vi "Initialize.vi"(0 "Universal Robot in":refnum<class "Universal Robot.lvclass">, 5 "error in (no error)":errorcluster) -> (14 "Universal Robot out":refnum<class "Universal Robot.lvclass">, 19 "error out":errorcluster)   [LabVIEW 2016, in "Universal Robot.lvclass"]
uses:
  Universal Robot.lvclass
  Universal Robot.lvclass/Universal Robot.ctl
  ProgramControlEvent.ctl
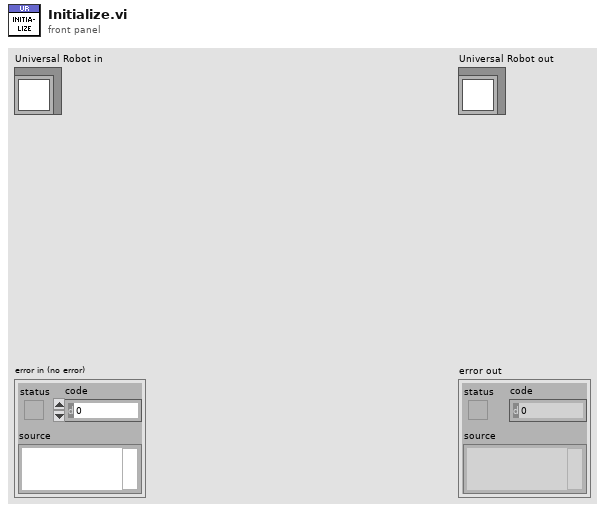
[diagram p1: front panel]
types:
  T1 = typedef "Universal Robot.lvclass/ProgramControlEvent.ctl" = enum16{"Stop", "Pause"}
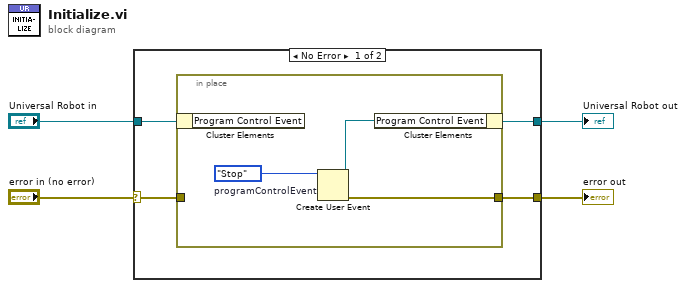
[diagram p0: block diagram]
diagram:
  n1 = case shown="No Error" "error in (no error)" {
    selector: "error in (no error)" -> [w8 w13]
    tunnel: [w7 w13] -> w3
    tunnel: [w5 w12] -> w1
    tunnel: "Universal Robot in" -> [w6 w12]
    frame No Error {
      n2 = in-place {
        in-place-border: w8 -> [_]
        in-place-border: [w9] -> w7
        w10 = ProgramControlEvent."Stop"  # programControlEvent
        n3 = in-place-cluster #1(w6) -> ()  [unwired: 1 out]
        n4 = Create User Event(user event datatype=w10) -> (user event=w11:refnum<user-event>, error out=w9:errorcluster)  [unwired: 1 in]
        n5 = in-place-cluster #1("Program Control Event"=w11) -> (w5:refnum<class "Universal Robot.lvclass">)
      }
    }
    frame Error {
    }
  }
  "error out" <- w3
  "Universal Robot out" <- w1
